vi "Example.vi"   [LabVIEW 2018]
uses:
  <vilib>/Skyline/TestMonitor/Shared/typedefs/Status Type.ctl
  7b21e067-cded-47bc-930e-c14918e6aaab.vi
  30d53454-e536-43d5-b4d6-289aa3c49ccd.vi
  <vilib>/Skyline/TestMonitor/Test Result/Create Test Result (Single).vi
  <vilib>/Skyline/JSON/Get Parameter Value (single).vi
  <vilib>/Skyline/TestMonitor/Named Value/Write Named Value.vi
  <vilib>/Skyline/TestMonitor/Test Step/Create Test Step (Single).vi
  <vilib>/Skyline/TestMonitor/Test Step/Update Test Step (Single).vi
  <vilib>/Skyline/TestMonitor/Test Result/Update Test Result (Single).vi
  <vilib>/Skyline/TestMonitor/Named Value/NI SystemLink Named Value.lvclass
  <vilib>/Skyline/TestMonitor/Test Result/NI SystemLink Test Result.lvclass
  <vilib>/Skyline/TestMonitor/Test Step/NI SystemLink Test Step.lvclass
  <vilib>/Skyline/Configuration/Configuration HTTP_class/Open Configuration HTTP Auto.vi
  <vilib>/Skyline/TestMonitor/Shared/NI SystemLink Test Monitor.lvlib
  <vilib>/Skyline/Configuration/Configuration_class/NI Skyline Configuration.lvclass
  <vilib>/Skyline/Configuration/Configuration HTTP_class/NI Skyline Configuration HTTP.lvclass
types:
  T1 = typedef "NI SystemLink Test Monitor.lvlib/Status Type.ctl" = enum16{"Failed", "Passed", "Looping", "Skipped", "Custom", "Done", "Running", "Waiting", "Terminated", "Errored", "Timed Out", "None"}
  T2 = cluster{"name":string, "measurement":dbl, "low limit":dbl, "high limit":dbl, "comparison type":string, "status":string, "units":string}
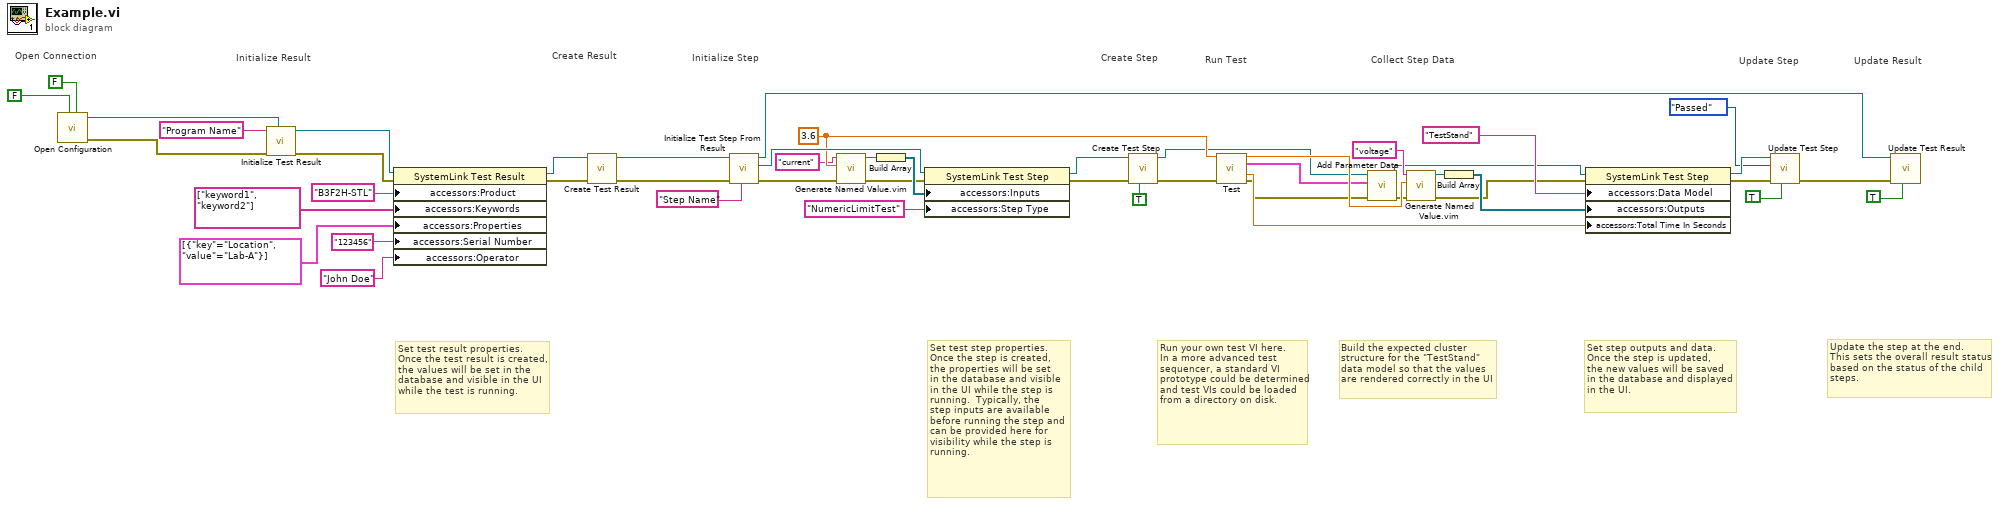
[diagram p0: block diagram]
diagram:
  w26 = 3.6
  # "Build the expected cluster\nstructure for the \"TestStand\"\ndata model so that the values\nare rendered correctly in the UI"
  # "Update the step at the end.\nThis sets the overall result status\nbased on the status of the child\nsteps."
  # "Set step outputs and data.\nOnce the step is updated,\nthe new values will be saved\nin the database and displayed\nin the UI."
  # "Set test step properties.\nOnce the step is created,\nthe properties will be set\nin the database and visible \nin the UI while the step is \nrunning.  Typically, the\nstep inputs are available\nbefore running the step and\ncan be provided here for\nvisibility while the step is\nrunning."
  # "Set test result properties.\nOnce the test result is created,\nthe values will be set in the\ndatabase and visible in the UI\nwhile the test is running."
  # "Update Result"
  # "Update Step"
  # "Collect Step Data"
  # "Run Test"
  # "Create Step"
  # "Initialize Step"
  # "Create Result"
  # "Initialize Result"
  # "Open Connection"
  # "Run your own test VI here.\nIn a more advanced test sequencer, a standard VI prototype could be determined and test VIs could be loaded from a directory on disk."
  n1 = call-poly <vilib>:"Open Configuration.vi"("HTTPS only?"=FALSE, "verify server?"=FALSE) -> ("error out"=w1:errorcluster, "configuration"=w2:refnum<class "NI Skyline Configuration HTTP.lvclass">)  [unwired: 8 in]
  n2 = call <vilib>:"Initialize Test Result.vi"("HTTP configuration"=w2, "error in (no error)"=w1, "program name"="Program Name") -> ("error out"=w46:errorcluster, "test result"=w47:refnum<class "NI SystemLink Test Result.lvclass">)  [unwired: 7 in]
  n3 = property class="SystemLink Test Result"(reference=w47, error in=w46, "accessors:Product"="B3F2H-STL" ("Product"), "accessors:Keywords"=string[] ["keyword1", "keyword2"] ("Keywords"), "accessors:Properties"=cluster{"key":string, "value":string}[] [{"key"="Location", "value"="Lab-A"}] ("Properties"), "accessors:Serial Number"="123456" ("Serial Number"), "accessors:Operator"="John Doe" ("Operator")) -> (reference out=w45:refnum<class "NI SystemLink Test Result.lvclass">, error out=w44:errorcluster)
  n4 = call-poly <vilib>:"Create Test Result.vi"("error in (no error)"=w44, "test result out"=w45) -> ("error out"=w41:errorcluster, "test result out"=w40:refnum<class "NI SystemLink Test Result.lvclass">)  [unwired: 8 in]
  n5 = call <vilib>:"Initialize Test Step From Result.vi"("step name"="Step Name", "error in (no error)"=w41, "test result in"=w40) -> ("error out"=w15:errorcluster, "test step"=w38:refnum<class "NI SystemLink Test Step.lvclass">, "test result out"=w9:refnum<class "NI SystemLink Test Result.lvclass">)  [unwired: 6 in]
  n6 = call "Generate Named Value.vim"("error in (no error)"=w15, "anything"=w26, "name"="current") -> ("error out"=w14:errorcluster, "named value"=w33:refnum<class "NI SystemLink Named Value.lvclass">)  [unwired: 7 in]
  n7 = Build Array(w33) -> (w32:refnum<class "NI SystemLink Named Value.lvclass">[])
  n8 = property class="SystemLink Test Step"(reference=w38, error in=w14, "accessors:Inputs"=w32, "accessors:Step Type"="NumericLimitTest" ("Step Type")) -> (reference out=w8:refnum<class "NI SystemLink Test Step.lvclass">, error out=w36:errorcluster)
  n9 = call-poly <vilib>:"Create Test Step.vi"("update result total time (F)"=TRUE, "error in (no error)"=w36, "test step in"=w8) -> ("error out"=w25:errorcluster, "test step out"=w6:refnum<class "NI SystemLink Test Step.lvclass">)  [unwired: 7 in]
  n10 = call "Test.vi"("current"=w26, "error in (no error)"=w25) -> ("voltage"=w30:dbl, "measurement data"=w7:T2, "test time"=w12:dbl, "error out"=w4:errorcluster)  [unwired: 10 in]
  n11 = call "Add Parameter Data.vi"("error in (no error)"=w4, "step parameters"=w7, "test step in"=w6) -> ("error out"=w3:errorcluster, "test step out"=w5:refnum<class "NI SystemLink Test Step.lvclass">)  [unwired: 7 in]
  n12 = call "Generate Named Value.vim"("error in (no error)"=w3, "anything"=w30, "name"="voltage") -> ("error out"=w13:errorcluster, "named value"=w28:refnum<class "NI SystemLink Named Value.lvclass">)  [unwired: 7 in]
  n13 = Build Array(w28) -> (w27:refnum<class "NI SystemLink Named Value.lvclass">[])
  n14 = property class="SystemLink Test Step"(reference=w5, error in=w13, "accessors:Data Model"="TestStand" ("Data Model"), "accessors:Outputs"=w27, "accessors:Total Time In Seconds"=w12) -> (reference out=w24:refnum<class "NI SystemLink Test Step.lvclass">, error out=w23:errorcluster)
  n15 = call-poly <vilib>:"Update Test Step.vi"("update result total time"=TRUE, "error in (no error)"=w23, "status type"=Status_Type."Passed", "test step in"=w24) -> ("error out"=w11:errorcluster)  [unwired: 6 in, 1 out]
  n16 = call-poly <vilib>:"Update Test Result.vi"("determine status from steps (F)"=TRUE, "error in (no error)"=w11, "test result in"=w9) -> ()  [unwired: 7 in, 2 out]
